vi "Flush Data to Log File.vi"(8 "error in (no error)":errorcluster, 10 "Data Queue":refnum<queue>, 11 "Logging Configuration 2":T1={"Log File Base Path"=path "", "TDMS File Reference"=refnum, "Log File Base Path 2"=path "C:/Users/J.Schwartz/Documents/LabVIEW Data/Space Station Test/Test Data/Test 1_2017_06_13_16_01_42.tdms", "TDMS File Reference 2"=refnum}) -> (0 "error out":errorcluster)   [LabVIEW 2018, in "System Logging.lvlib" / "Logging.lvlib"]
doc: "Flush the data queue of any pending data and write it to the log file. Close the TDMS file reference."
uses:
  Logging.lvlib
  <vilib>/Waveform/WDTOps.llb/WDT Get Waveform Time Array DBL.vi
  Logging Configuration.ctl
panel:
  out "remaining elements":cluster{"Array":waveform(dbl)[]}[](array[cluster])
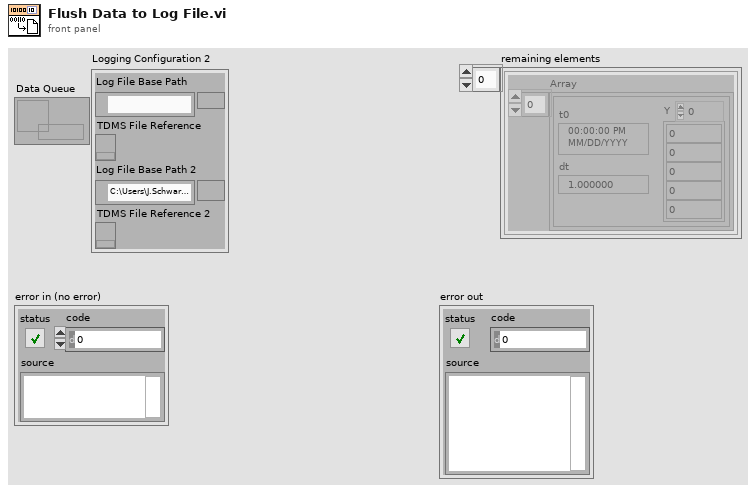
[diagram p1: front panel]
types:
  T1 = typedef "System Logging.lvlib/Logging.lvlib/Logging Configuration.ctl" = cluster{"Log File Base Path":path, "TDMS File Reference":refnum<k34>, "Log File Base Path 2":path, "TDMS File Reference 2":refnum<k34>}
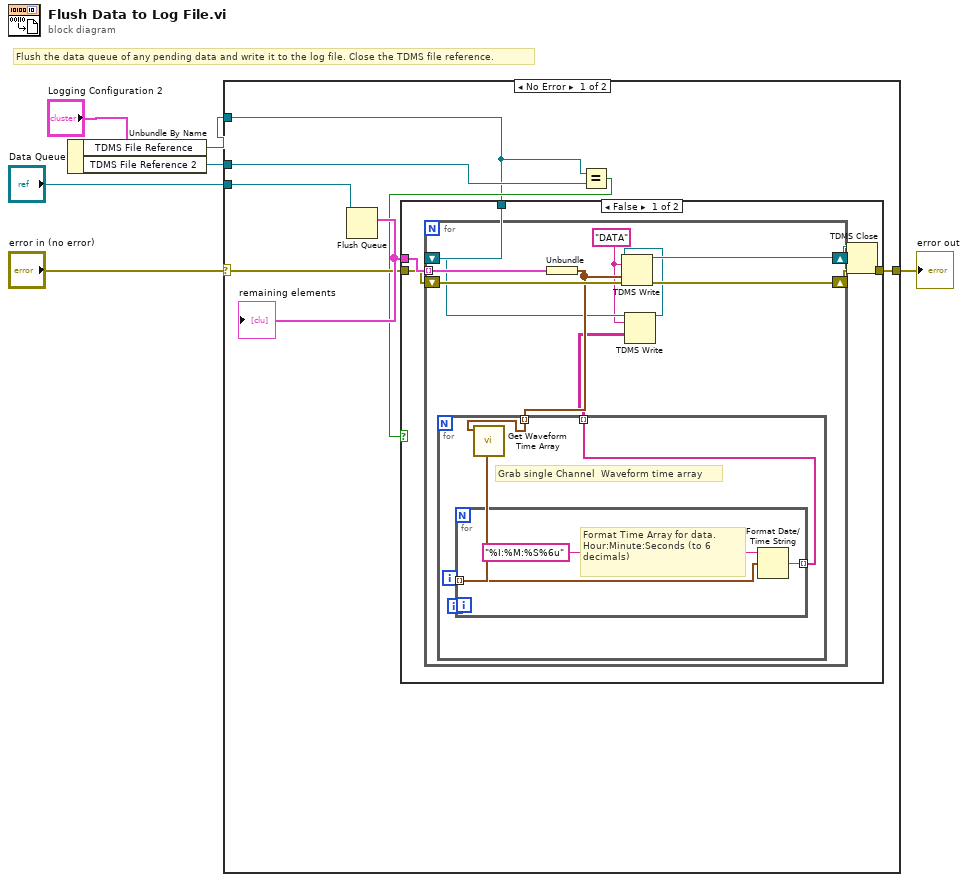
[diagram p0: block diagram]
diagram:
  # "Flush the data queue of any pending data and write it to the log file. Close the TDMS file reference."
  n1 = Unbundle By Name("Logging Configuration 2") -> ("TDMS File Reference"=w2:refnum<k34>, "TDMS File Reference 2"=w1:refnum<k34>)
  n2 = case shown="No Error" "error in (no error)" {
    selector: "error in (no error)" -> [w10 w36]
    tunnel: "Data Queue" -> [w12 _]
    tunnel: [w11 w36] -> w5
    tunnel: w2 -> [w7 _]
    tunnel: w1 -> [w9 _]
    frame No Error {
      n3 = Flush Queue(queue=w12) -> (remaining elements=w13:cluster{"Array":waveform(dbl)[]}[])  [unwired: 1 in, 2 out]
      "remaining elements" <- w13
      n4 = Equal?(x=w7, y=w9) -> (x = y?=w8:bool)
      n5 = case shown="False" w8 {
        tunnel: w13 -> [w19 _]
        tunnel: [w17 w35] -> w11
        tunnel: w10 -> [w16 w35]
        tunnel: w7 -> [w14 _]
        frame False {
          n6 = for {
            shift-right: [w26] -> w15
            shift-left: w14 -> [w23]
            shift-right: [w27] -> w18
            shift-left: w16 -> [w28]
            tunnel: w19 -> [w25] mode=indexing
            w21 = "DATA" ("group name in (Untitled)")
            n7 = Unbundle(w25) -> ("Array"=w24:waveform(dbl)[])
            n8 = for {
              tunnel: w24 -> [w31] mode=indexing
              tunnel: [w29] -> w20 mode=indexing
              # "Grab single Channel  Waveform time array"
              n9 = call-poly <vilib>:"Get Waveform Time Array.vi"("waveform in"=w31) -> ("X array"=w30:timestamp[])  [unwired: 9 in, 1 out]
              n10 = for {
                tunnel: w30 -> [w34] mode=indexing
                tunnel: [w33] -> w29 mode=indexing
                # "Format Time Array for data. Hour:Minute:Seconds (to 6 decimals)"
                n11 = Format Date/Time String(time format string (%c)="%I:%M:%S%6u", seconds (now)=w34) -> (date/time string=w33:string)  [unwired: 1 in]
              }
            }
            n12 = TDMS Write(0:w23, 5:w21, 9:w20) -> (4:w22:refnum<k34>)  [unwired: 3 in, 3 out]
            n13 = TDMS Write(0:w22, 5:w21, 9:w24, 11:w28) -> (4:w26:refnum<k34>, 15:w27:errorcluster)  [unwired: 2 in, 2 out]
          }
          n14 = TDMS Close(8:w18, 11:w15) -> (0:w17:errorcluster)  [unwired: 1 out]
        }
        frame True {
        }
      }
    }
    frame Error {
    }
  }
  "error out" <- w5
